vi "Initiate Multipart Upload.vi"(4 "Region":T1, 7 "Request Parameters":T3={"Content Type"="binary/octet-stream", "ACL"=enum."private", "Storage Class"=enum."STANDARD", "User Metadata"=[]}, 8 "error in (no error)":errorcluster, 9 "Bucket":string, 10 "Object Path":string) -> (0 "error out":errorcluster, 3 "Multipart Upload RefNum":T2)   [LabVIEW 2015, in "LV Interface for Amazon S3.lvlib"]
doc: "This operation <B>initiates a multipart upload</B> operation and <B>returns a Multipart Upload Refnum</B>. <B>After</B> initiating a multipart upload process, <B>you can start uploading the individual parts</B> of the object. Multipart uploads provide the following advantages: <B> - Improved throughput</B>: You can upload parts in parallel to improve throughput. <B> - Quick recovery from any network issues</B>: Smaller part size minimizes the impact of restarting a failed upload due to a network error. <B> - Pause and resume object uploads</B>: You can upload object parts over time. Once you initiate a multipart upload there is no expiry; you must explicitly complete or abort the multipart upload. <B> - Begin an upload before you know the final object size</B>: You can upload an object as you are creating it."
uses:
  LV Interface for Amazon S3.lvlib
  Typedefs/AMZ_S3_API_POST Multipart Object Request Parameters.ctl
  Typedefs/AMZ_S3_ACL.ctl
  Typedefs/AMZ_S3_Storage Class.ctl
  Typedefs/AMZ_S3_Object Metadata.ctl
  Typedefs/AMZ_S3_Multipart Upload RefNum.ctl
  Typedefs/AMZ_S3_Multipart Upload RefNum Enum.ctl
  Typedefs/AMZ_S3_LocationConstraint.ctl
  Typedefs/AMZ_S3_Multipart Upload Data.ctl
  Typedefs/AMZ_S3_Multipart Upload Part Data.ctl
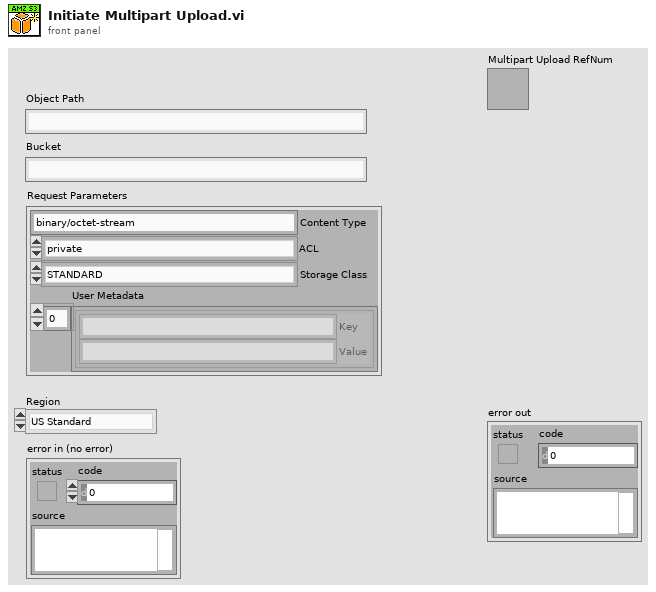
[diagram p1: front panel]
types:
  T1 = typedef "LV Interface for Amazon S3.lvlib/AMZ_S3_LocationConstraint.ctl" = enum16{"US Standard", "us-east-2", "us-west-1", "us-west-2", "ap-northeast-1", "ap-northeast-2", "ap-southeast-1", "ap-southeast-2", "ca-central-1", "eu-central-1", "eu-west-1", "eu-west-2", "sa-east-1"}
  T2 = typedef "LV Interface for Amazon S3.lvlib/AMZ_S3_Multipart Upload RefNum.ctl" = refnum<k1>
  T3 = typedef "LV Interface for Amazon S3.lvlib/AMZ_S3_API_POST Multipart Object Request Parameters.ctl" = cluster{"Content Type":string, "ACL":T4, "Storage Class":T5, "User Metadata":T6[]}
  T4 = typedef "LV Interface for Amazon S3.lvlib/AMZ_S3_ACL.ctl" = enum16{"private", "public-read", "public-read-write", "aws-exec-read", "authenticated-read", "bucket-owner-read", "bucket-owner-full-control"}
  T5 = typedef "LV Interface for Amazon S3.lvlib/AMZ_S3_Storage Class.ctl" = enum16{"STANDARD", "REDUCED_REDUNDANCY"}
  T6 = typedef "LV Interface for Amazon S3.lvlib/AMZ_S3_Object Metadata.ctl" = cluster{"Key":string, "Value":string}
  T7 = typedef "LV Interface for Amazon S3.lvlib/AMZ_S3_HTTP Header-Value pair.ctl" = cluster{"Header":string, "Value":string}
  T8 = typedef "LV Interface for Amazon S3.lvlib/AMZ_S3_Call Results.ctl" = enum16{"Success", "UndefinedError", "AccessDenied", "AccountProblem", "AmbiguousGrantByEmailAddress", "BadDigest", "BucketAlreadyExists", "BucketAlreadyOwnedByYou", "BucketNotEmpty", "CredentialsNotSupported", "CrossLocationLoggingProhibited", "EntityTooSmall", "EntityTooLarge", "ExpiredToken", "IllegalVersioningConfigurationException", "IncompleteBody", "IncorrectNumberOfFilesInPostRequest", "InlineDataTooLarge", "InternalError", "InvalidAccessKeyId", "InvalidAddressingHeader", "InvalidArgument", "InvalidBucketName", "InvalidDigest", "InvalidLocationConstraint", "InvalidPart", "InvalidPartOrder", "InvalidPayer", "InvalidPolicyDocument", "InvalidRange", "InvalidSecurity", "InvalidSOAPRequest", "InvalidStorageClass", "InvalidTargetBucketForLogging", "InvalidToken", "InvalidURI", "KeyTooLong", "MalformedACLError", "MalformedPOSTRequest", "MalformedXML", "MaxMessageLengthExceeded", "MaxPostPreDataLengthExceededError", "MetadataTooLarge", "MethodNotAllowed", "MissingAttachment", "MissingContentLength", "MissingRequestBodyError", "MissingSecurityElement", "MissingSecurityHeader", "NoLoggingStatusForKey", "NoSuchBucket", "NoSuchKey", "NoSuchUpload", "NoSuchVersion", "NotImplemented", "NotSignedUp", "OperationAborted", "PermanentRedirect", "PreconditionFailed", "Redirect", "RequestIsNotMultiPartContent", "RequestTimeout", "RequestTimeTooSkewed", "RequestTorrentOfBucketError", "SignatureDoesNotMatch", "SlowDown", "TemporaryRedirect", "TokenRefreshRequired", "TooManyBuckets", "UnexpectedContent", "UnresolvableGrantByEmailAddress", "UserKeyMustBeSpecified", "LabVIEWError"}
  T9 = typedef "LV Interface for Amazon S3.lvlib/AMZ_S3_Multipart Upload Data.ctl" = cluster{"Object":string, "Bucket":string, "UploadID":string, "Parts":T10[]}
  T10 = typedef "LV Interface for Amazon S3.lvlib/AMZ_S3_Multipart Upload Part Data.ctl" = cluster{"PartNumber":u16, "Lat modified":timestamp, "ETag":string, "Size":u64}
  T11 = typedef "LV Interface for Amazon S3.lvlib/AMZ_S3_API_InitiateMultipartUploadResult.ctl" = cluster{"Bucket":string, "Key":string, "UploadID":string}
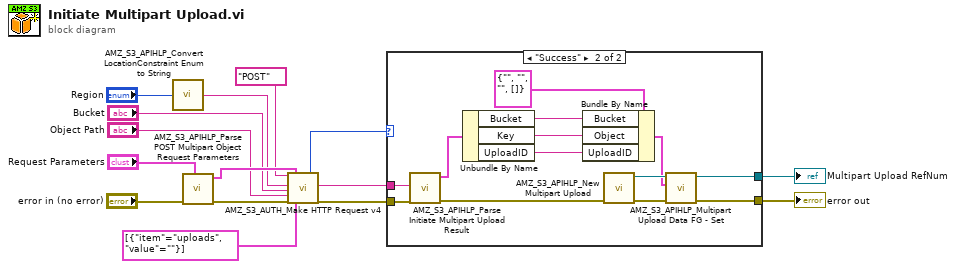
[diagram p0: block diagram]
diagram:
  n1 = call "AMZ_S3_APIHLP_Convert LocationConstraint Enum to String.vi"("Location"="Region") -> ("Location String"=w1:string)  [unwired: 4 in]
  n2 = call "AMZ_S3_APIHLP_Parse POST Multipart Object Request Parameters.vi"("POST Multipart Object Request Parameters"="Request Parameters", "error in (no error)"="error in (no error)") -> ("error out"=w11:errorcluster, "HTTP Headers"=w7:T7[])  [unwired: 8 in]
  n3 = call "AMZ_S3_AUTH_Make HTTP Request v4.vi"("HTTP-Verb"="POST", "Region"=w1, "Bucket"="Bucket", "Object Key"="Object Path", "error in"=w11, "request headers"=w7, "request parameters"=cluster{"item":string, "value":string}[] [{"item"="uploads", "value"=""}]) -> ("Call Result"=w9:T8, "response body"=w8:string, "error out"=w10:errorcluster)  [unwired: 9 in, 1 out]
  n4 = case shown="\"Success\"" w9 {
    tunnel: w10 -> [w16 w29]
    tunnel: [w16 w19] -> w13
    tunnel: [_ w18] -> w12
    tunnel: w8 -> [_ w17]
    frame Default {
    }
    frame "Success" {
      n5 = call "AMZ_S3_APIHLP_Parse Initiate Multipart Upload Result.vi"("error in (no error)"=w29, "Response body"=w17) -> ("error out"=w28:errorcluster, "InitiateMultipartUploadResult"=w25:T11)  [unwired: 8 in]
      n6 = Unbundle By Name(w25) -> ("Bucket"=w22:string, "Key"=w23:string, "UploadID"=w21:string)
      n7 = Bundle By Name(cluster=T9 {"Object"="", "Bucket"="", "UploadID"="", "Parts"=[]} ("Multipart Upload Data"), "Bucket"=w22, "Object"=w23, "UploadID"=w21) -> (w20:T9)
      n8 = call "AMZ_S3_APIHLP_New Multipart Upload.vi"("error in (no error)"=w28) -> ("error out"=w27:errorcluster, "Multipart Upload RefNum"=w26:T2)  [unwired: 9 in]
      n9 = call "AMZ_S3_APIHLP_Multipart Upload Data FG - Set.vi"("error in (no error)"=w27, "Multipart Upload Data"=w20, "Multipart Upload RefNum in"=w26) -> ("error out"=w19:errorcluster, "Multipart Upload RefNum out"=w18:T2)  [unwired: 6 in, 1 out]
    }
  }
  "error out" <- w13
  "Multipart Upload RefNum" <- w12
